vi "util_create_config.vi"(8 "error in (no error)":errorcluster, 9 "config_value":T2, 10 "config_include":T1, 11 "config_file in":path) -> (0 "error out":errorcluster, 3 "config_file out":path)   [LabVIEW 2015, in "lv-bin-7zip.lvlib"]
uses:
  lv-bin-7zip.lvlib
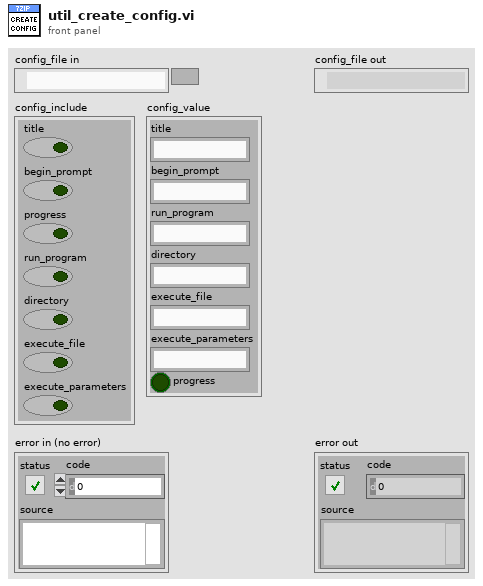
[diagram p1: front panel]
types:
  T1 = cluster{"title":bool, "begin_prompt":bool, "progress":bool, "run_program":bool, "directory":bool, "execute_file":bool, "execute_parameters":bool}
  T2 = cluster{"title":string, "begin_prompt":string, "run_program":string, "directory":string, "execute_file":string, "execute_parameters":string, "progress":bool}
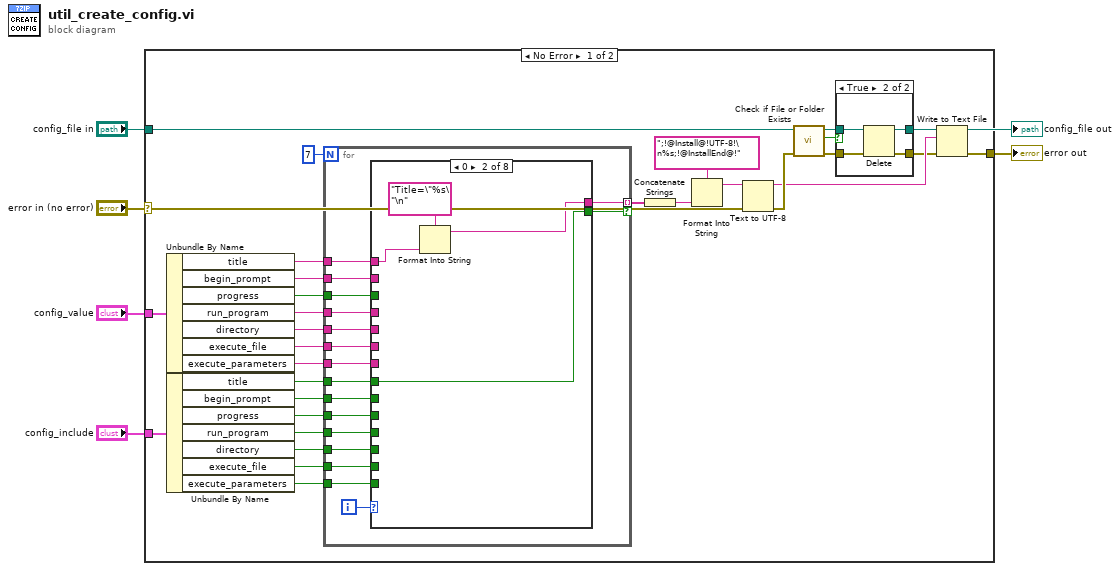
[diagram p0: block diagram]
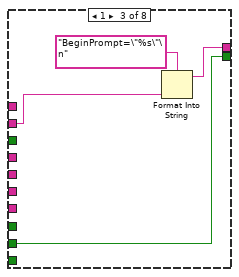
[diagram p3: hidden frame]
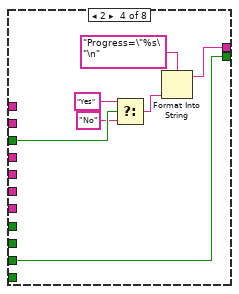
[diagram p4: hidden frame]
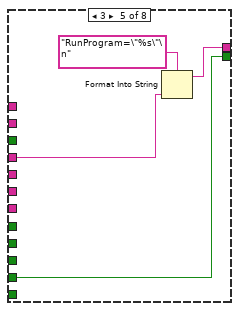
[diagram p5: hidden frame]
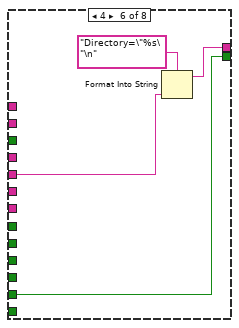
[diagram p6: hidden frame]
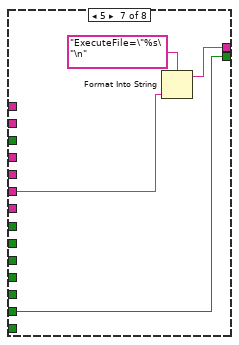
[diagram p7: hidden frame]
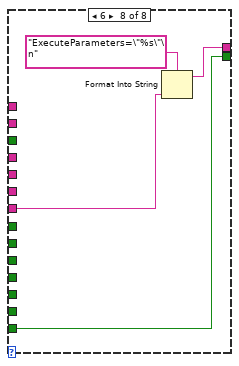
[diagram p8: hidden frame]
diagram:
  n1 = case shown="No Error" "error in (no error)" {
    selector: "error in (no error)" -> [w6 w91]
    tunnel: [w29 w91] -> w5
    tunnel: "config_value" -> [w28 _]
    tunnel: "config_file in" -> [w7 _]
    tunnel: "config_include" -> [w20 _]
    frame No Error {
      n2 = Unbundle By Name(w28) -> ("title"=w27:string, "begin_prompt"=w26:string, "progress"=w25:bool, "run_program"=w24:string, "directory"=w23:string, "execute_file"=w22:string, "execute_parameters"=w21:string)
      n3 = Unbundle By Name(w20) -> ("title"=w19:bool, "begin_prompt"=w18:bool, "progress"=w17:bool, "run_program"=w16:bool, "directory"=w15:bool, "execute_file"=w14:bool, "execute_parameters"=w13:bool)
      n4 = for {
        N: 7 -> [_]
        tunnel: w27 -> [w46]
        tunnel: w26 -> [w47]
        tunnel: w25 -> [w48]
        tunnel: w24 -> [w49]
        tunnel: w23 -> [w50]
        tunnel: w22 -> [w51]
        tunnel: w21 -> [w52]
        tunnel: w19 -> [w45]
        tunnel: w18 -> [w44]
        tunnel: w17 -> [w43]
        tunnel: w16 -> [w42]
        tunnel: w15 -> [w41]
        tunnel: w14 -> [w40]
        tunnel: w13 -> [w39]
        tunnel: [w38] -> w12 mode=indexing if=w37
        i -> [w53]
        n5 = case shown="0" w53 {
          tunnel: w52 -> [_ _ _ _ _ _ _ w82]
          tunnel: w51 -> [_ _ _ _ _ _ w78 _]
          tunnel: w50 -> [_ _ _ _ _ w74 _ _]
          tunnel: w49 -> [_ _ _ _ w70 _ _ _]
          tunnel: w48 -> [_ _ _ w66 _ _ _ _]
          tunnel: w47 -> [_ _ w58 _ _ _ _ _]
          tunnel: w46 -> [_ w56 _ _ _ _ _ _]
          tunnel: w45 -> [_ w55 _ _ _ _ _ _]
          tunnel: w44 -> [_ _ w59 _ _ _ _ _]
          tunnel: w43 -> [_ _ _ w65 _ _ _ _]
          tunnel: w42 -> [_ _ _ _ w69 _ _ _]
          tunnel: w41 -> [_ _ _ _ _ w73 _ _]
          tunnel: w40 -> [_ _ _ _ _ _ w77 _]
          tunnel: w39 -> [_ _ _ _ _ _ _ w81]
          tunnel: [_ w54 w60 w67 w71 w75 w79 w83] -> w38
          tunnel: [_ w55 w59 w65 w69 w73 w77 w81] -> w37
          frame Default {
          }
          frame 0 {
            n6 = Format Into String(format string="Title=\"%s\"\n", w56) -> (resulting string=w54:string)  [unwired: 2 in, 1 out]
          }
          frame 1 {
            n7 = Format Into String(format string="BeginPrompt=\"%s\"\n", w58) -> (resulting string=w60:string)  [unwired: 2 in, 1 out]
          }
          frame 2 {
            n8 = Select(t="Yes", s=w66, f="No") -> (s? t:f=w62:string)
            n9 = Format Into String(format string="Progress=\"%s\"\n", w62) -> (resulting string=w67:string)  [unwired: 2 in, 1 out]
          }
          frame 3 {
            n10 = Format Into String(format string="RunProgram=\"%s\"\n", w70) -> (resulting string=w71:string)  [unwired: 2 in, 1 out]
          }
          frame 4 {
            n11 = Format Into String(format string="Directory=\"%s\"\n", w74) -> (resulting string=w75:string)  [unwired: 2 in, 1 out]
          }
          frame 5 {
            n12 = Format Into String(format string="ExecuteFile=\"%s\"\n", w78) -> (resulting string=w79:string)  [unwired: 2 in, 1 out]
          }
          frame 6 {
            n13 = Format Into String(format string="ExecuteParameters=\"%s\"\n", w82) -> (resulting string=w83:string)  [unwired: 2 in, 1 out]
          }
        }
      }
      n14 = Concatenate Strings(w12) -> (w11:string)
      n15 = Format Into String(format string=";!@Install@!UTF-8!\n%s;!@InstallEnd@!", w11) -> (resulting string=w9:string)  [unwired: 2 in, 1 out]
      n16 = Text to UTF-8(8:w6, 11:w9) -> (0:w36:errorcluster, 3:w35:string)  [unwired: 1 in]
      n17 = call <vilib>:"Check if File or Folder Exists.vi"("error in (no error)"=w36, "path"=w7) -> ("error out"=w33:errorcluster, "file or folder exists?"=w34:bool, "dup path"=w32:path)  [unwired: 7 in]
      n18 = case shown="True" w34 {
        tunnel: w33 -> [w85 w90]
        tunnel: w32 -> [w86 w89]
        tunnel: [w86 w88] -> w31
        tunnel: [w85 w87] -> w30
        frame False {
        }
        frame True {
          n19 = Delete(path (use dialog)=w89, error in=w90) -> (deleted path=w88:path, error out=w87:errorcluster)  [unwired: 3 in, 1 out]
        }
      }
      n20 = Write to Text File(file (use dialog)=w31, text=w35, error in=w30) -> (error out=w29:errorcluster)  [unwired: 1 in, 2 out]
    }
    frame Error {
    }
  }
  "error out" <- w5
  "config_file out" <- "config_file in"
